vi "Trim string both ends to just alphanum.vi"(8 "error in (no error)":errorcluster, 11 "string":string) -> (0 "error out":errorcluster, 3 "String out":string)   [LabVIEW 2013]
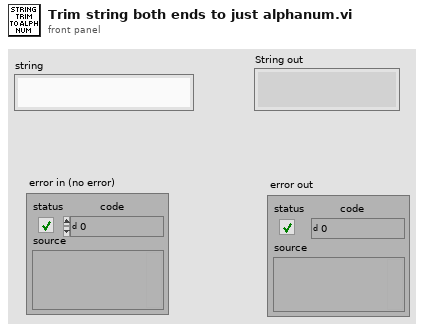
[diagram p1: front panel]
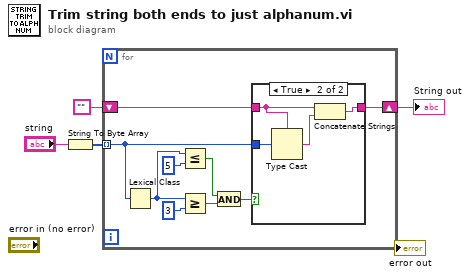
[diagram p0: block diagram]
diagram:
  n1 = String To Byte Array(string="string") -> (unsigned byte array=w3:u8[])
  n2 = for {
    tunnel: w3 -> [w9] mode=indexing
    shift-right: [w10] -> w1
    shift-left: "" -> [w11]
    n3 = Lexical Class(1:w9) -> (0:w5:i16)
    n4 = Less Or Equal?(x=w5, y=u8 5) -> (x <= y?=w7:bool)
    n5 = Greater Or Equal?(x=w5, y=i16 3) -> (x >= y?=w8:bool)
    n6 = And(x=w7, y=w8) -> (x .and. y?=w6:bool)
    n7 = case shown="True" w6 {
      tunnel: w11 -> [w14 w16]
      tunnel: [w14 w18] -> w10
      tunnel: w9 -> [_ w17]
      frame False {
      }
      frame True {
        n8 = Type Cast(type=w16, x=w17) -> (*(type *) &x=w15:string)
        n9 = Concatenate Strings(w16, w15) -> (w18:string)
      }
    }
  }
  "String out" <- w1
